vi "Get Result.vi"(8 "error in (no error)":errorcluster, 11 "Simple VISA Reader Driver in":refnum<class "Simple VISA Reader Driver.lvclass">) -> (0 "error out":errorcluster, 2 "Result":refnum<class "Acquired Result.lvclass">, 3 "Simple VISA Reader Driver out":refnum<class "Simple VISA Reader Driver.lvclass">)   [LabVIEW 2016, in "Simple VISA Reader Driver.lvclass"]
uses:
  Simple VISA Reader Driver.lvclass
  C:/github/NHMFL_Core/Libraries/Instruments/Instrument Driver/Instrument Driver.lvclass
  LabActor/Results/Acquired Result/Acquired Result.lvclass
  Instrument Driver/Instrument Driver.lvclass/Instrument Driver.ctl
  LabActor/Results/Acquired Result/Acquired Result.lvclass/Acquired Result.ctl
  Instrument Driver/Read Channel names.vi
  Instrument Driver/Read Group name.vi
  Instrument Driver/Read Channel units.vi
  LabActor/Results/Acquired Result/Write Channels.vi
  LabActor/Results/Acquired Result/Write Group.vi
  <vilib>/express/express shared/transition.llb/Dynamic To Waveform Array.vi
  <vilib>/express/express signal manip/GetorSetDDTAttributes/Set DDT Attributes/SetT0.vi
  <vilib>/express/express shared/transition.llb/Waveform Array To Dynamic.vi
  <vilib>/express/express signal manip/GetorSetDDTAttributes/Set DDT Attributes/Set DDT Properties.xnode
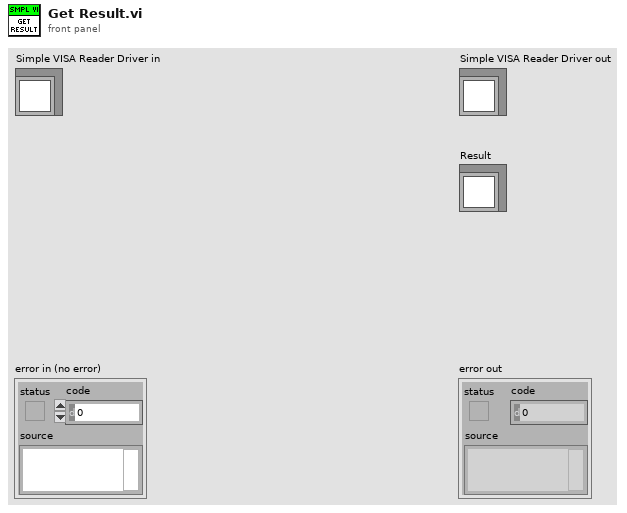
[diagram p1: front panel]
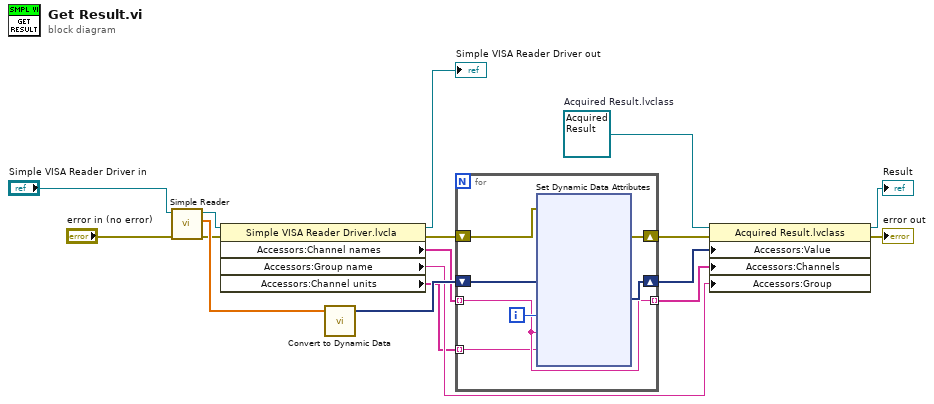
[diagram p0: block diagram]
diagram:
  w15 = refnum<class "Acquired Result.lvclass"> refnum  # Acquired Result.lvclass
  n1 = call-dynamic "Simple Reader.vi"("error in (no error)"="error in (no error)", "Simple VISA Reader Driver in"="Simple VISA Reader Driver in") -> ("error out"=w5:errorcluster, "Signals"=w10:dbl[], "Simple VISA Reader Driver out"=w7:refnum<class "Simple VISA Reader Driver.lvclass">)  [unwired: 7 in]
  n2 = property class="Simple VISA Reader Driver.lvcla"(reference=w7, error in=w5) -> (reference out=→"Simple VISA Reader Driver out":refnum<class "Simple VISA Reader Driver.lvclass">, error out=w1:errorcluster, "Accessors:Channel names"=w4:string[], "Accessors:Group name"=w3:string, "Accessors:Channel units"=w2:string[])
  n3 = call "Convert to Dynamic Data"("Array"=w10) -> ("Dynamic Data Type"=w16:dynamicdata)  [unwired: 3 in]
  n4 = for {
    tunnel: [w19] -> w13 mode=indexing
    tunnel: w4 -> [w19] mode=indexing
    tunnel: w2 -> [w18] mode=indexing
    shift-right: [w21] -> w17
    shift-left: w16 -> [w22]
    shift-right: [w23] -> w14
    shift-left: w1 -> [w24]
    i -> [w20]
    n5 = xnode "Set Dynamic Data Attributes"("Signals In"=w22, "Signal Index"=w20, "Signal Name"=w19, "Unit"=w18, "error in"=w24) -> ("Signals Out"=w21:dynamicdata, "error out"=w23:errorcluster)
  }
  n6 = property class="Acquired Result.lvclass"(reference=w15, error in=w14, "Accessors:Value"=w17, "Accessors:Channels"=w13, "Accessors:Group"=w3) -> (reference out=→"Result":refnum<class "Acquired Result.lvclass">, error out=→"error out":errorcluster)
